vi "update CVT values thorlabsWFS.vi"(5 "Refnum in 2":T1, 7 "Array":bool[](array[boolean]), 8 "error in (no error)":errorcluster, 9 "output cluster":dbl[](array[numeric]), 10 "ZernikeCoeffs":sgl[](array[numeric]), 11 "Refnum in":T1) -> (0 "error out":errorcluster)   [LabVIEW 2020, in "ThorlabsWFS.lvclass"]
uses:
  ThorlabsWFS.lvclass
  IMAQ Image.ctl
  GUIcompressionCluster.ctl
  OnOffTypeDef.ctl
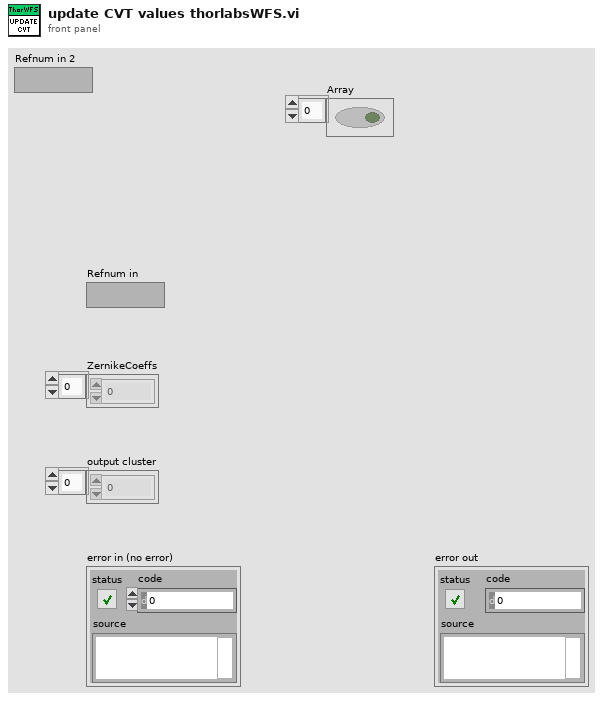
[diagram p1: front panel]
types:
  T1 = typedef "IMAQ Image.ctl" = refnum<image>
  T2 = typedef "GUIcompressionCluster.ctl" = cluster{"GUI8bit":T3, "GUICompression":T3, "CompressionQuality":i32}
  T3 = typedef "OnOffTypeDef.ctl" = enum16{"off", "on"}
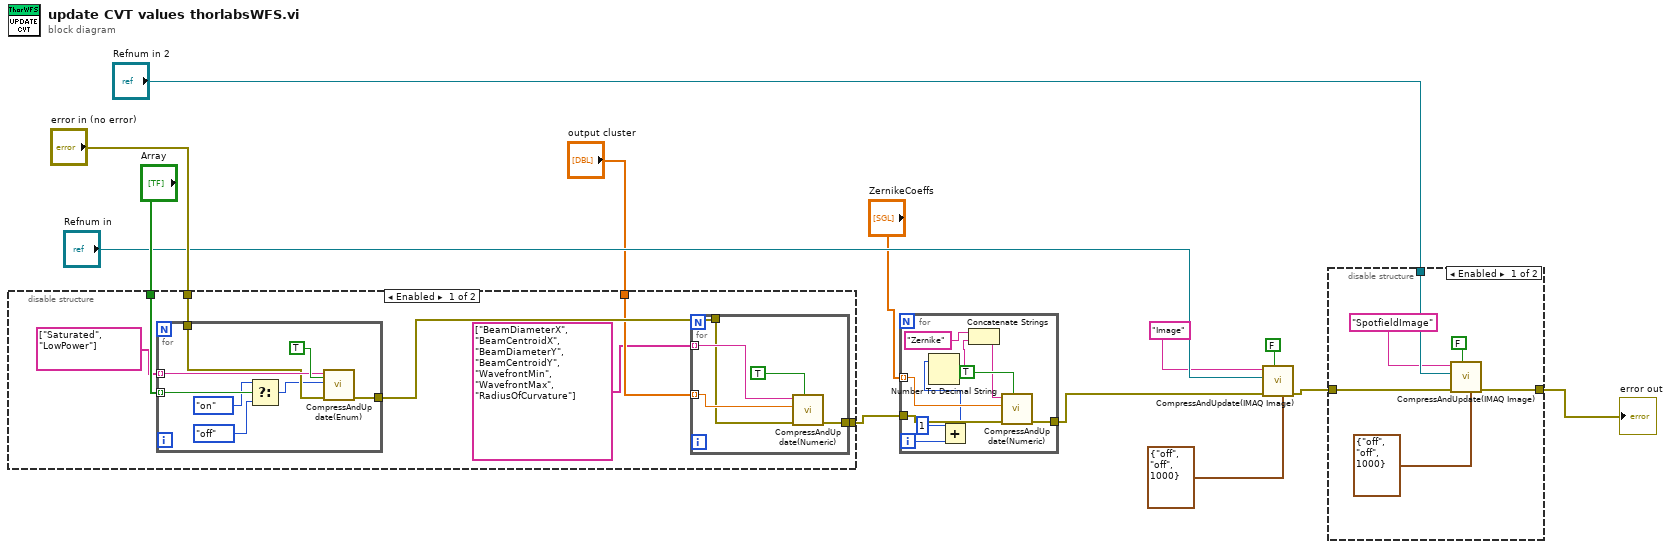
[diagram p0: block diagram]
diagram:
  n1 = disable-structure shown="Enabled" {
    disable-tunnel: "error in (no error)" -> [w19 w34]
    disable-tunnel: "Array" -> [w18 _]
    disable-tunnel: [w16 w34] -> w6
    disable-tunnel: "output cluster" -> [w15 _]
    frame Enabled {
      n2 = for {
        tunnel: string[] ["Saturated", "LowPower"] -> [w27] mode=indexing
        tunnel: w18 -> [w24] mode=indexing
        tunnel: w19 -> [w26]
        tunnel: [w25] -> w20
        n3 = Select(t=OnOffTypeDef."on" ("Settings.Trigger"), s=w24, f=OnOffTypeDef."off" ("Settings.Trigger")) -> (s? t:f=w21:T3)
        n4 = call "CompressAndUpdate(Enum).vi"("force CVT update (false)"=TRUE, "error in"=w26, "enum variant"=w21, "command or variable name"=w27) -> ("error out"=w25:errorcluster)  [unwired: 7 in]
      }
      n5 = for {
        tunnel: string[] ["BeamDiameterX", "BeamCentroidX", "BeamDiameterY", "BeamCentroidY", "WavefrontMin", "WavefrontMax", "RadiusOfCurvature"] -> [w32] mode=indexing
        tunnel: w15 -> [w31] mode=indexing
        tunnel: w20 -> [w30]
        tunnel: [w29] -> w16
        n6 = call "CompressAndUpdate(Numeric).vi"("force CVT update (false)"=TRUE, "error in"=w30, "Numeric"=w31, "command or variable name"=w32) -> ("error out"=w29:errorcluster)  [unwired: 7 in]
      }
    }
    frame Disabled {
    }
  }
  n7 = for {
    tunnel: [w43] -> w5
    tunnel: w6 -> [w39]
    tunnel: "ZernikeCoeffs" -> [w38] mode=indexing
    i -> [w37]
    n8 = Add(x=1, y=w37) -> (x+y=w35:i32)
    n9 = Number To Decimal String(number=w35) -> (decimal integer string=w41:string)  [unwired: 1 in]
    n10 = Concatenate Strings("Zernike" ("command or variable name"), w41) -> (w40:string)
    n11 = call "CompressAndUpdate(Numeric).vi"("force CVT update (false)"=TRUE, "error in"=w39, "Numeric"=w38, "command or variable name"=w40) -> ("error out"=w43:errorcluster)  [unwired: 7 in]
  }
  n12 = call "CompressAndUpdate(IMAQ Image).vi"("GUICompression"=T2 {"GUI8bit"=enum."off", "GUICompression"=enum."off", "CompressionQuality"=1000}, "force CVT update (false)"=FALSE, "error in"=w5, "IMAQ Image"="Refnum in", "command or variable name"="Image") -> ("error out"=w8:errorcluster)  [unwired: 6 in]
  n13 = disable-structure shown="Enabled" {
    disable-tunnel: "Refnum in 2" -> [w50 _]
    disable-tunnel: w8 -> [w49 _]
    disable-tunnel: [w45 _] -> w4
    frame Enabled {
      n14 = call "CompressAndUpdate(IMAQ Image).vi"("GUICompression"=T2 {"GUI8bit"=enum."off", "GUICompression"=enum."off", "CompressionQuality"=1000}, "force CVT update (false)"=FALSE, "error in"=w49, "IMAQ Image"=w50, "command or variable name"="SpotfieldImage") -> ("error out"=w45:errorcluster)  [unwired: 6 in]
    }
    frame Disabled {
    }
  }
  "error out" <- w4
